vi "Init RxTx.vi"(8 "error in (no error)":errorcluster, 11 "Channel in":refnum<class "Channel.lvclass">) -> (0 "error out":errorcluster, 3 "Channel out":refnum<class "Channel.lvclass">)   [LabVIEW 2018, in "Channel.lvclass"]
uses:
  Channel.lvclass
  Channel.lvclass/Channel.ctl
  RxTx/RxTx.lvclass
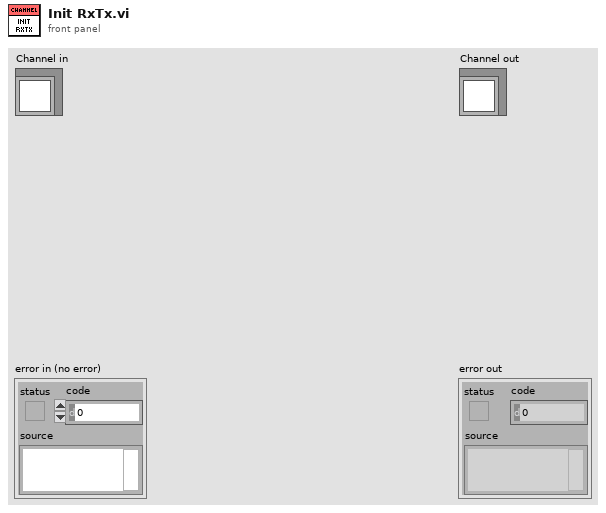
[diagram p1: front panel]
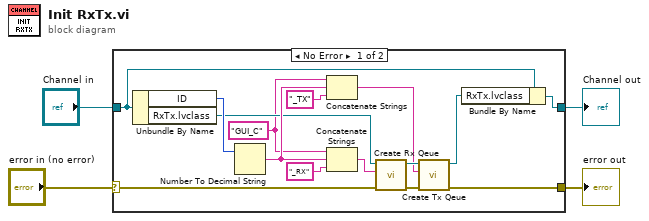
[diagram p0: block diagram]
diagram:
  n1 = case shown="No Error" "error in (no error)" {
    selector: "error in (no error)" -> [w13 w21]
    tunnel: [w10 w21] -> w2
    tunnel: [w18 w20] -> w1
    tunnel: "Channel in" -> [w19 w20]
    frame No Error {
      w5 = "GUI_C"
      n2 = Unbundle By Name(w19) -> ("ID"=w14:u16, "RxTx.lvclass"=w12:refnum<class "RxTx.lvclass">)
      n3 = Number To Decimal String(number=w14) -> (decimal integer string=w15:string)  [unwired: 1 in]
      n4 = Concatenate Strings(w5, w15, "_TX") -> (w7:string)
      n5 = Concatenate Strings(w5, w15, "_RX") -> (w11:string)
      n6 = call "Create Rx Qeue.vi"("error in (no error)"=w13, "Reader Name"=w11, "RxTx in"=w12) -> ("error out"=w6:errorcluster, "RxTx out"=w8:refnum<class "RxTx.lvclass">)  [unwired: 7 in]
      n7 = call "Create Tx Qeue.vi"("error in (no error)"=w6, "Writer Name"=w7, "RxTx in"=w8) -> ("error out"=w10:errorcluster, "RxTx out"=w9:refnum<class "RxTx.lvclass">)  [unwired: 7 in]
      n8 = Bundle By Name(cluster=w19, "RxTx.lvclass"=w9) -> (w18:refnum<class "Channel.lvclass">)
    }
    frame Error {
    }
  }
  "error out" <- w2
  "Channel out" <- w1
